vi "ex14-6.vi"() -> ()   [LabVIEW 2014]
uses:
  <vilib>/NXT/Subs/MotorOutput.ctl
  <vilib>/NXT/Dual Mode Library/prims/inRangeAndCoerce/inRangeAndCoerce_float.vi
  <vilib>/NXT/Dual Mode Library/Motors/MotorDistance_Single.vi
panel:
  out "負數或溢位?65536\n[減法]":bool
  in  "X":dbl
  in  "Y":dbl
  in  "SUB":bool
  out "X-Y":dbl
  out "X+Y":dbl
  out "負數或溢位?65536\n[加法]":bool
  in  "ADD":bool
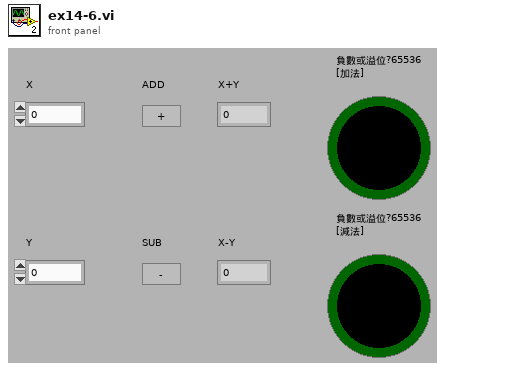
[diagram p1: front panel]
types:
  T1 = typedef "MotorOutput.ctl" = u8
  T2 = typedef "LVHSConnector.ctl" = refnum<class "BrickReference.lvclass">
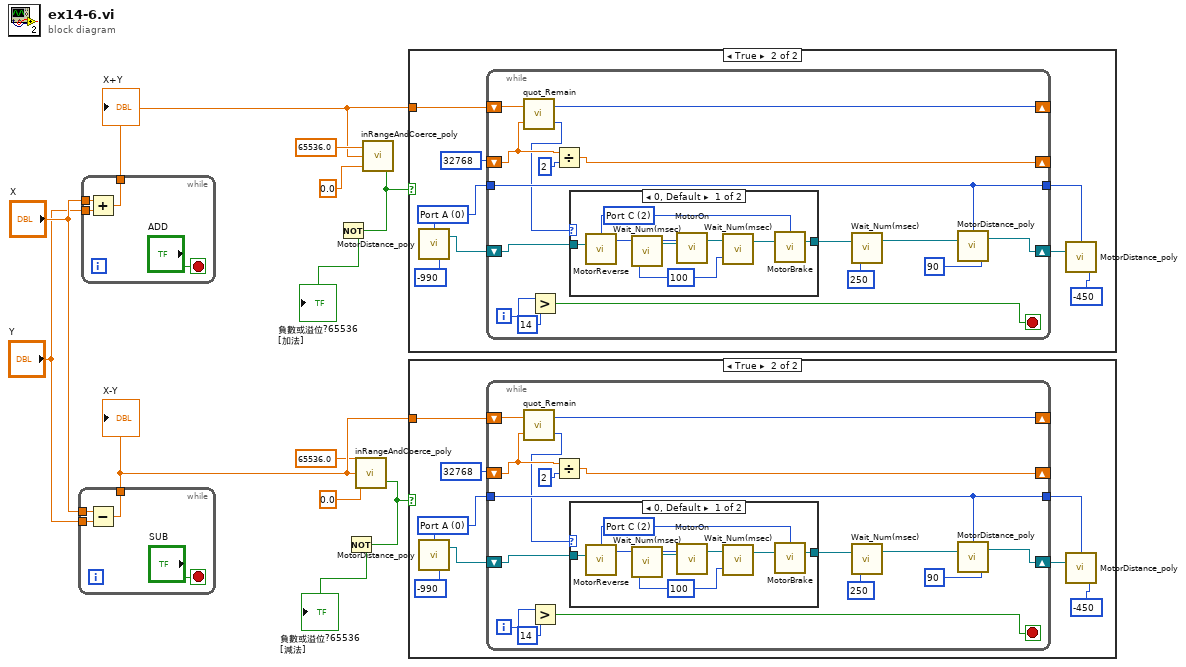
[diagram p0: block diagram]
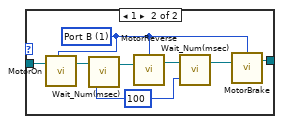
[diagram p3: hidden frame]
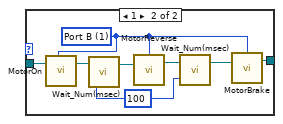
[diagram p5: hidden frame]
diagram:
  n1 = while {
    tunnel: [w15] -> w8
    tunnel: "X" -> [w14]
    tunnel: "Y" -> [w13]
    stop <- "SUB" stop-if-true
    n2 = Subtract(x=w14, y=w13) -> (x-y=w15:dbl)
  }
  "X-Y" <- w8
  n3 = while {
    tunnel: [w19] -> w1
    tunnel: "X" -> [w18]
    tunnel: "Y" -> [w17]
    stop <- "ADD" stop-if-true
    n4 = Add(x=w18, y=w17) -> (x+y=w19:dbl)
  }
  "X+Y" <- w1
  n5 = call-poly <vilib>:"inRangeAndCoerce_poly.vi"("lower limit"=0.0 ("y"), "x"=w8, "upper limit"=65536.0 ("y")) -> ("In Range?"=w5:bool)  [unwired: 1 out]
  n6 = Not(x=w5) -> (.not. x?=→"負數或溢位?65536\n[減法]":bool)
  n7 = call-poly <vilib>:"inRangeAndCoerce_poly.vi"("lower limit"=0.0 ("y"), "x"=w1, "upper limit"=65536.0 ("y")) -> ("In Range?"=w2:bool)  [unwired: 1 out]
  n8 = Not(x=w2) -> (.not. x?=→"負數或溢位?65536\n[加法]":bool)
  n9 = case shown="True" w2 {
    tunnel: w1 -> [_ w21]
    frame False {
    }
    frame True {
      w23 = T1 0 items=["Port A", "Port B", "Port C", "All Ports"] ("Output Port (All Ports)")
      n10 = call-poly <vilib>:"MotorDistance_poly.vi"("Angle of Rotation (360)"=-990 ("Distance (100)"), "Output Port (All Ports)"=w23) -> ("NXT/EV3"=w26:T2)  [unwired: 2 in]
      n11 = while {
        shift-right: [w30] -> _
        shift-left: w21 -> [w32]
        shift-right: [w43] -> _
        shift-left: 32768 -> [w31]
        shift-right: [w36] -> w25
        shift-left: w26 -> [w42]
        tunnel: w23 -> [w37]
        tunnel: [w37] -> w22
        i -> [w41]
        stop <- w39 stop-if-true
        n12 = call <vilib>:"quot_Remain.vi"("y"=w31, "x"=w32) -> ("floor(x/y)"=w29:i32, "x-y*floor(x/y)"=w30:i32)
        n13 = Greater?(x=w41, y=14) -> (0:w39:bool)
        n14 = Divide(x=w31, y=2) -> (x/y=w43:dbl)
        n15 = case shown="0, Default" w29 {
          tunnel: w42 -> [w48 w55]
          tunnel: [w49 w54] -> w35
          frame 0, Default {
            w50 = u32 100 ("Time (100 msec)")
            w52 = T1 2 items=["Port A", "Port B", "Port C", "All Ports"] ("Output Port (All Ports)")
            n16 = call <vilib>:"MotorReverse.vi"("NXT/EV3"=w48, "Output Port (All Ports)"=w52) -> ("NXT/EV3"=w47:T2)  [unwired: 2 in]
            n17 = call <vilib>:"Wait_Num(msec).vi"("Time (100 msec)"=w50, "NXT/EV3"=w47) -> ("NXT/EV3"=w46:T2)  [unwired: 2 in]
            n18 = call <vilib>:"MotorOn.vi"("NXT/EV3"=w46, "Output Port (All Ports)"=w52) -> ("NXT/EV3"=w45:T2)  [unwired: 2 in]
            n19 = call <vilib>:"Wait_Num(msec).vi"("Time (100 msec)"=w50, "NXT/EV3"=w45) -> ("NXT/EV3"=w51:T2)  [unwired: 2 in]
            n20 = call <vilib>:"MotorBrake.vi"("NXT/EV3"=w51, "Port (All Ports)"=w52) -> ("NXT/EV3"=w49:T2)  [unwired: 2 in]
          }
          frame 1 {
            w53 = u32 100 ("Time (100 msec)")
            w60 = T1 1 items=["Port A", "Port B", "Port C", "All Ports"] ("Output Port (All Ports)")
            n21 = call <vilib>:"MotorOn.vi"("NXT/EV3"=w55, "Output Port (All Ports)"=w60) -> ("NXT/EV3"=w56:T2)  [unwired: 2 in]
            n22 = call <vilib>:"Wait_Num(msec).vi"("Time (100 msec)"=w53, "NXT/EV3"=w56) -> ("NXT/EV3"=w57:T2)  [unwired: 2 in]
            n23 = call <vilib>:"MotorReverse.vi"("NXT/EV3"=w57, "Output Port (All Ports)"=w60) -> ("NXT/EV3"=w58:T2)  [unwired: 2 in]
            n24 = call <vilib>:"Wait_Num(msec).vi"("Time (100 msec)"=w53, "NXT/EV3"=w58) -> ("NXT/EV3"=w59:T2)  [unwired: 2 in]
            n25 = call <vilib>:"MotorBrake.vi"("NXT/EV3"=w59, "Port (All Ports)"=w60) -> ("NXT/EV3"=w54:T2)  [unwired: 2 in]
          }
        }
        n26 = call <vilib>:"Wait_Num(msec).vi"("Time (100 msec)"=u32 250, "NXT/EV3"=w35) -> ("NXT/EV3"=w34:T2)  [unwired: 2 in]
        n27 = call-poly <vilib>:"MotorDistance_poly.vi"("Angle of Rotation (360)"=90 ("Distance (100)"), "NXT/EV3"=w34, "Output Port (All Ports)"=w37) -> ("NXT/EV3"=w36:T2)  [unwired: 1 in]
      }
      n28 = call-poly <vilib>:"MotorDistance_poly.vi"("Angle of Rotation (360)"=-450 ("Distance (100)"), "NXT/EV3"=w25, "Output Port (All Ports)"=w22) -> ()  [unwired: 1 in, 1 out]
    }
  }
  n29 = case shown="True" w5 {
    tunnel: w8 -> [_ w61]
    frame False {
    }
    frame True {
      w63 = T1 0 items=["Port A", "Port B", "Port C", "All Ports"] ("Output Port (All Ports)")
      n30 = call-poly <vilib>:"MotorDistance_poly.vi"("Angle of Rotation (360)"=-990 ("Distance (100)"), "Output Port (All Ports)"=w63) -> ("NXT/EV3"=w66:T2)  [unwired: 2 in]
      n31 = while {
        shift-right: [w70] -> _
        shift-left: w61 -> [w72]
        shift-right: [w83] -> _
        shift-left: 32768 -> [w71]
        shift-right: [w76] -> w65
        shift-left: w66 -> [w82]
        tunnel: w63 -> [w77]
        tunnel: [w77] -> w62
        i -> [w81]
        stop <- w79 stop-if-true
        n32 = call <vilib>:"quot_Remain.vi"("y"=w71, "x"=w72) -> ("floor(x/y)"=w69:i32, "x-y*floor(x/y)"=w70:i32)
        n33 = Greater?(x=w81, y=14) -> (0:w79:bool)
        n34 = Divide(x=w71, y=2) -> (x/y=w83:dbl)
        n35 = case shown="0, Default" w69 {
          tunnel: w82 -> [w88 w95]
          tunnel: [w89 w94] -> w75
          frame 0, Default {
            w90 = u32 100 ("Time (100 msec)")
            w92 = T1 2 items=["Port A", "Port B", "Port C", "All Ports"] ("Output Port (All Ports)")
            n36 = call <vilib>:"MotorReverse.vi"("NXT/EV3"=w88, "Output Port (All Ports)"=w92) -> ("NXT/EV3"=w87:T2)  [unwired: 2 in]
            n37 = call <vilib>:"Wait_Num(msec).vi"("Time (100 msec)"=w90, "NXT/EV3"=w87) -> ("NXT/EV3"=w86:T2)  [unwired: 2 in]
            n38 = call <vilib>:"MotorOn.vi"("NXT/EV3"=w86, "Output Port (All Ports)"=w92) -> ("NXT/EV3"=w85:T2)  [unwired: 2 in]
            n39 = call <vilib>:"Wait_Num(msec).vi"("Time (100 msec)"=w90, "NXT/EV3"=w85) -> ("NXT/EV3"=w91:T2)  [unwired: 2 in]
            n40 = call <vilib>:"MotorBrake.vi"("NXT/EV3"=w91, "Port (All Ports)"=w92) -> ("NXT/EV3"=w89:T2)  [unwired: 2 in]
          }
          frame 1 {
            w93 = u32 100 ("Time (100 msec)")
            w100 = T1 1 items=["Port A", "Port B", "Port C", "All Ports"] ("Output Port (All Ports)")
            n41 = call <vilib>:"MotorOn.vi"("NXT/EV3"=w95, "Output Port (All Ports)"=w100) -> ("NXT/EV3"=w96:T2)  [unwired: 2 in]
            n42 = call <vilib>:"Wait_Num(msec).vi"("Time (100 msec)"=w93, "NXT/EV3"=w96) -> ("NXT/EV3"=w97:T2)  [unwired: 2 in]
            n43 = call <vilib>:"MotorReverse.vi"("NXT/EV3"=w97, "Output Port (All Ports)"=w100) -> ("NXT/EV3"=w98:T2)  [unwired: 2 in]
            n44 = call <vilib>:"Wait_Num(msec).vi"("Time (100 msec)"=w93, "NXT/EV3"=w98) -> ("NXT/EV3"=w99:T2)  [unwired: 2 in]
            n45 = call <vilib>:"MotorBrake.vi"("NXT/EV3"=w99, "Port (All Ports)"=w100) -> ("NXT/EV3"=w94:T2)  [unwired: 2 in]
          }
        }
        n46 = call <vilib>:"Wait_Num(msec).vi"("Time (100 msec)"=u32 250, "NXT/EV3"=w75) -> ("NXT/EV3"=w74:T2)  [unwired: 2 in]
        n47 = call-poly <vilib>:"MotorDistance_poly.vi"("Angle of Rotation (360)"=90 ("Distance (100)"), "NXT/EV3"=w74, "Output Port (All Ports)"=w77) -> ("NXT/EV3"=w76:T2)  [unwired: 1 in]
      }
      n48 = call-poly <vilib>:"MotorDistance_poly.vi"("Angle of Rotation (360)"=-450 ("Distance (100)"), "NXT/EV3"=w65, "Output Port (All Ports)"=w62) -> ()  [unwired: 1 in, 1 out]
    }
  }
